vi "insert_block.vi"(5 "repetition":i32=1 min=1, 6 "start pixel coordinate":T1, 7 "mode":T2, 8 "error in (no error)":errorcluster, 10 "block":refnum<class "Image.lvclass">, 11 "Image in":refnum<class "Image.lvclass">) -> (0 "error out":errorcluster, 3 "Image out":refnum<class "Image.lvclass">)   [LabVIEW 2010, in "Image.lvclass"]
uses:
  Image.lvclass
  insert_mode_enum.ctl
  clusters/pixel_coordinate_cluster.ctl
  storage_mode.ctl
  ErrorController/ErrorController/class_data.vi
  <vilib>/vision/NI_Vision_Development_Module.lvlib
  ErrorController/ErrorController/ErrorController.lvclass
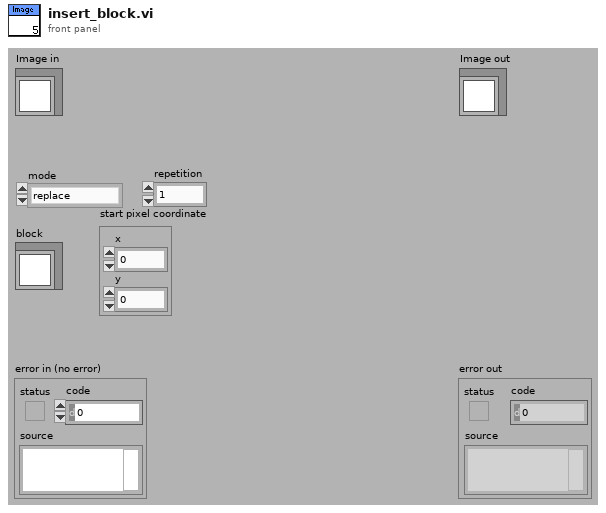
[diagram p1: front panel]
types:
  T1 = typedef "pixel_coordinate_cluster.ctl" = cluster{"x":i32, "y":i32}
  T2 = typedef "Image.lvclass/insert_mode_enum.ctl" = enum16{"replace", "average"}
  T3 = typedef "Image.lvclass/storage_mode.ctl" = enum16{"RAM", "disk"}
  T4 = typedef "IMAQ Image.ctl" = refnum<image>
  T5 = typedef "Image Type" = u32
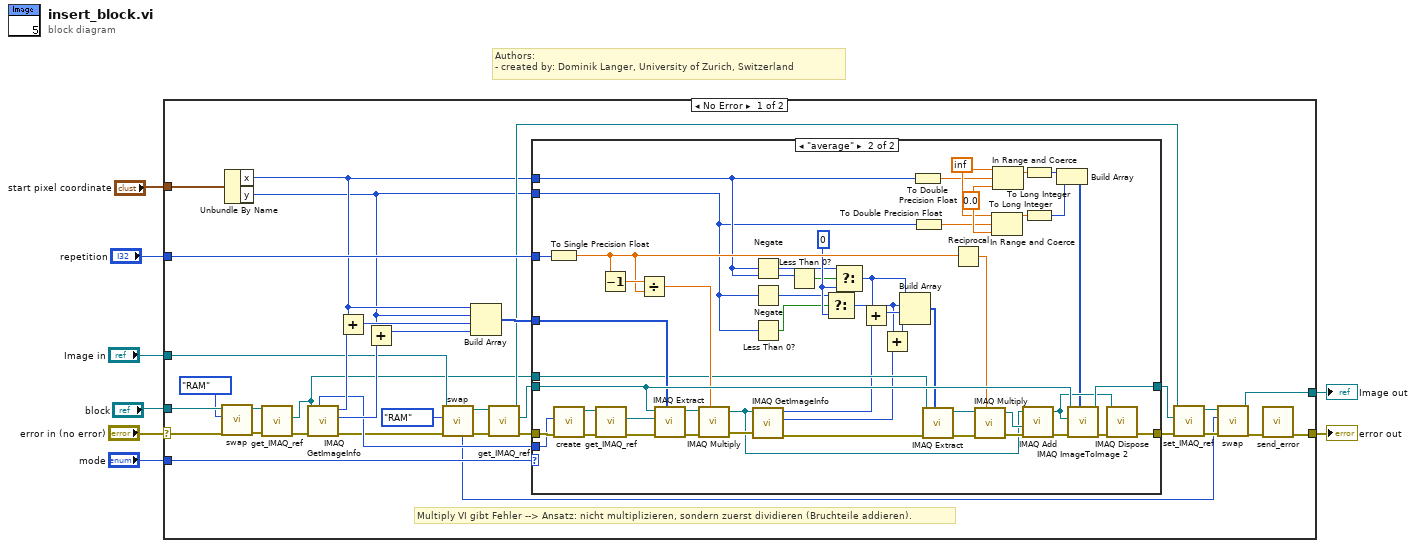
[diagram p0: block diagram]
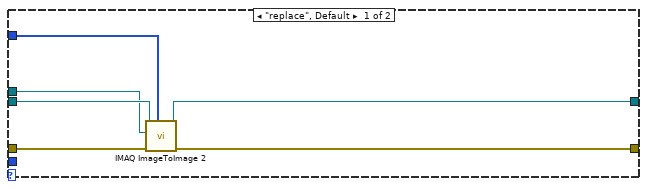
[diagram p2: hidden frame]
diagram:
  # "Authors: \n- created by: Dominik Langer, University of Zurich, Switzerland"
  n1 = case shown="No Error" "error in (no error)" {
    selector: "error in (no error)" -> [w18 w101]
    tunnel: [w9 w101] -> w7
    tunnel: [w27 w100] -> w5
    tunnel: "Image in" -> [w24 w100]
    tunnel: "mode" -> [w42 _]
    tunnel: "block" -> [w17 _]
    tunnel: "repetition" -> [w40 _]
    tunnel: "start pixel coordinate" -> [w13 _]
    frame No Error {
      # "Multiply VI gibt Fehler --> Ansatz: nicht multiplizieren, sondern zuerst dividieren (Bruchteile addieren)."
      n2 = call-dynamic "swap.vi"("error in (no error)"=w18, "storage type target"=storage_mode."RAM", "Image in"=w17) -> ("error out"=w16:errorcluster, "Image out"=w15:refnum<class "Image.lvclass">)  [unwired: 7 out]
      n3 = Unbundle By Name(w13) -> ("x"=w12:i32, "y"=w11:i32)
      n4 = call-dynamic "get_IMAQ_ref.vi"("error in (no error)"=w16, "Image.lvclass in"=w15) -> ("error out"=w20:errorcluster, "Image"=w19:T4)  [unwired: 8 out]
      n5 = call "IMAQ GetImageInfo"("error in (no error)"=w20, "Image"=w19) -> ("error out"=w26:errorcluster, "Y Resolution"=w34:i32, "X Resolution"=w35:i32, "Image Type"=w33:T5)  [unwired: 6 out]
      n6 = Add(x=w12, y=w35) -> (x+y=w39:i32)
      n7 = Add(x=w11, y=w34) -> (x+y=w38:i32)
      n8 = call-dynamic "swap.vi"("error in (no error)"=w26, "storage type target"=storage_mode."RAM", "Image in"=w24) -> ("error out"=w25:errorcluster, "Image out"=w23:refnum<class "Image.lvclass">, "previous storage mode"=w22:T3)  [unwired: 6 out]
      n9 = Build Array(w12, w11, w39, w38) -> (w41:i32[])
      n10 = call-dynamic "get_IMAQ_ref.vi"("error in (no error)"=w25, "Image.lvclass in"=w23) -> ("error out"=w37:errorcluster, "Image"=w36:T4, "Image.lvclass out"=w30:refnum<class "Image.lvclass">)  [unwired: 7 out]
      n11 = case shown="\"average\"" w42 {
        tunnel: w36 -> [w48 w93]
        tunnel: w37 -> [w47 w83]
        tunnel: w19 -> [w46 w71]
        tunnel: [w45 w95] -> w31
        tunnel: [w44 w90] -> w32
        tunnel: w41 -> [w43 w92]
        tunnel: w40 -> [_ w94]
        tunnel: w33 -> [_ w82]
        tunnel: w12 -> [_ w63]
        tunnel: w11 -> [_ w61]
        frame "replace", Default {
          n12 = call "IMAQ ImageToImage 2"("Offset Left/Top"=w43, "error in (no error)"=w47, "Image Src (Small)"=w46, "Image Src (Large)"=w48) -> ("error out"=w44:errorcluster, "Image Dst Out"=w45:T4)  [unwired: 2 in, 4 out]
        }
        frame "average" {
          w64 = inf
          w65 = 0.0 ("lower limit")
          w72 = 0
          n13 = To Single Precision Float(number=w94) -> (single precision float=w86:sgl)
          n14 = call "create.vi"("error in (no error)"=w83, "Image Type"=w82) -> ("error out"=w81:errorcluster, "Image out"=w80:refnum<class "Image.lvclass">)  [unwired: 2 in, 6 out]
          n15 = call-dynamic "get_IMAQ_ref.vi"("error in (no error)"=w81, "Image.lvclass in"=w80) -> ("error out"=w79:errorcluster, "Image"=w78:T4)  [unwired: 8 out]
          n16 = Decrement(x=w86) -> (x-1=w88:sgl)
          n17 = Divide(x=w88, y=w86) -> (x/y=w87:sgl)
          n18 = call "IMAQ Extract"("Optional Rectangle"=w92, "error in (no error)"=w79, "Image Dst"=w78, "Image Src"=w93) -> ("error out"=w99:errorcluster, "Image Dst Out"=w97:T4)  [unwired: 2 in, 4 out]
          n19 = call "IMAQ Multiply"("Image Src A"=w97, "Constant"=w87, "error in (no error)"=w99) -> ("Image Dst Out"=w76:T4, "error out"=w77:errorcluster)  [unwired: 2 in, 2 out]
          n20 = Negate(x=w63) -> (-x=w70:i32)
          n21 = Negate(x=w61) -> (-x=w69:i32)
          n22 = Less Than 0?(x=w61) -> (x < 0?=w67:bool)
          n23 = call "IMAQ GetImageInfo"("error in (no error)"=w77, "Image"=w76) -> ("error out"=w55:errorcluster, "Y Resolution"=w49:i32, "X Resolution"=w54:i32)  [unwired: 7 out]
          n24 = Less Than 0?(x=w63) -> (x < 0?=w68:bool)
          n25 = Select(t=w69, s=w67, f=w72) -> (s? t:f=w51:i32)
          n26 = Select(t=w70, s=w68, f=w72) -> (s? t:f=w52:i32)
          n27 = Add(x=w52, y=w54) -> (x+y=w53:i32)
          n28 = Add(x=w51, y=w49) -> (x+y=w50:i32)
          n29 = Build Array(w52, w51, w53, w50) -> (w73:i32[])
          n30 = To Double Precision Float(number=w63) -> (double precision float=w62:dbl)
          n31 = To Double Precision Float(number=w61) -> (double precision float=w60:dbl)
          n32 = call "IMAQ Extract"("Optional Rectangle"=w73, "error in (no error)"=w55, "Image Src"=w71) -> ("error out"=w75:errorcluster, "Image Dst Out"=w74:T4)  [unwired: 3 in, 4 out]
          n33 = Reciprocal(x=w86) -> (1/x=w85:sgl)
          n34 = call "IMAQ Multiply"("Image Src A"=w74, "Constant"=w85, "error in (no error)"=w75) -> ("Image Dst Out"=w84:T4, "error out"=w98:errorcluster)  [unwired: 2 in, 2 out]
          n35 = In Range and Coerce(upper limit=w64, x=w60, lower limit=w65) -> (coerced(x)=w59:dbl)  [unwired: 1 out]
          n36 = In Range and Coerce(upper limit=w64, x=w62, lower limit=w65) -> (coerced(x)=w57:dbl)  [unwired: 1 out]
          n37 = call "IMAQ Add"("Image Src A"=w76, "Image Src B"=w84, "error in (no error)"=w98) -> ("Image Dst Out"=w89:T4, "error out"=w96:errorcluster)  [unwired: 2 in, 2 out]
          n38 = To Long Integer(number=w57) -> (32bit integer=w56:i32)
          n39 = To Long Integer(number=w59) -> (32bit integer=w58:i32)
          n40 = Build Array(w56, w58) -> (w66:i32[])
          n41 = call "IMAQ ImageToImage 2"("Offset Left/Top"=w66, "error in (no error)"=w96, "Image Src (Small)"=w89, "Image Src (Large)"=w93) -> ("error out"=w91:errorcluster, "Image Dst Out"=w95:T4)  [unwired: 2 in, 4 out]
          n42 = call "IMAQ Dispose"("Image"=w89, "error in (no error)"=w91) -> ("error out"=w90:errorcluster)  [unwired: 1 in, 3 out]
        }
      }
      n43 = call-dynamic "set_IMAQ_ref.vi"("error in (no error)"=w32, "Image"=w31, "Image.lvclass in"=w30) -> ("error out"=w29:errorcluster, "Image.lvclass out"=w28:refnum<class "Image.lvclass">)  [unwired: 7 out]
      n44 = call-dynamic "swap.vi"("error in (no error)"=w29, "storage type target"=w22, "Image in"=w28) -> ("error out"=w10:errorcluster, "Image out"=w27:refnum<class "Image.lvclass">)  [unwired: 7 out]
      n45 = call "send_error.vi"("error in (no error)"=w10) -> ("error out"=w9:errorcluster)  [unwired: 10 in]
    }
    frame Error {
    }
  }
  "error out" <- w7
  "Image out" <- w5
